vi "IsRead.vi"(6 "error in":errorcluster, 9 "Local in":refnum<class "Local.lvclass">) -> (0 "error out":errorcluster, 2 "is read":bool, 3 "Local out":refnum<class "Local.lvclass">)   [LabVIEW 2014, in "Raspberry Pi Compatible Compiler for LabVIEW.lvlib" / "Local.lvclass"]
uses:
  Local.lvclass
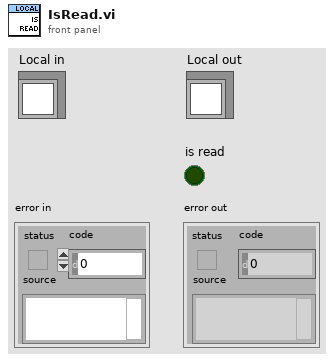
[diagram p1: front panel]
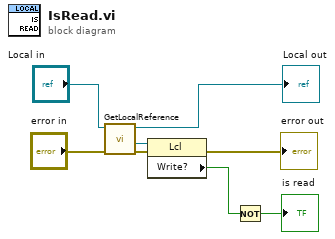
[diagram p0: block diagram]
diagram:
  n1 = call "GetLocalReference.vi"("error in"="error in", "Local in"="Local in") -> ("error out"=w5:errorcluster, "reference out"=w4:refnum<vi>, "Local out"=→"Local out":refnum<class "Local.lvclass">)  [unwired: 7 in]
  n2 = property class="Lcl"(reference=w4, error in=w5) -> (error out=→"error out":errorcluster, "Write?"=w1:bool)  [unwired: 1 out]
  n3 = Not(x=w1) -> (.not. x?=→"is read":bool)
